vi "Load AFM Subpanel.vi"(0 "Ring in":refnum<vi>, 1 "Background Image":refnum<vi>, 3 "name or relative path":string, 5 "Inkscape File (.svg)":refnum<vi>, 7 "input cluster":T2, 9 "Subpanel":refnum<vi>, 11 "error in (no error)":errorcluster, 12 "Run":refnum<vi>, 14 "Abort":refnum<vi>) -> (6 "reference out":refnum<vi>, 15 "error out":errorcluster)   [LabVIEW 2013]
doc: "This VI opens an AFM subpanel."
uses:
  <vilib>/Analysis/Matrix/Datatypes/RealMatrix.ctl
  <vilib>/Analysis/Matrix/NI_Matrix.lvlib
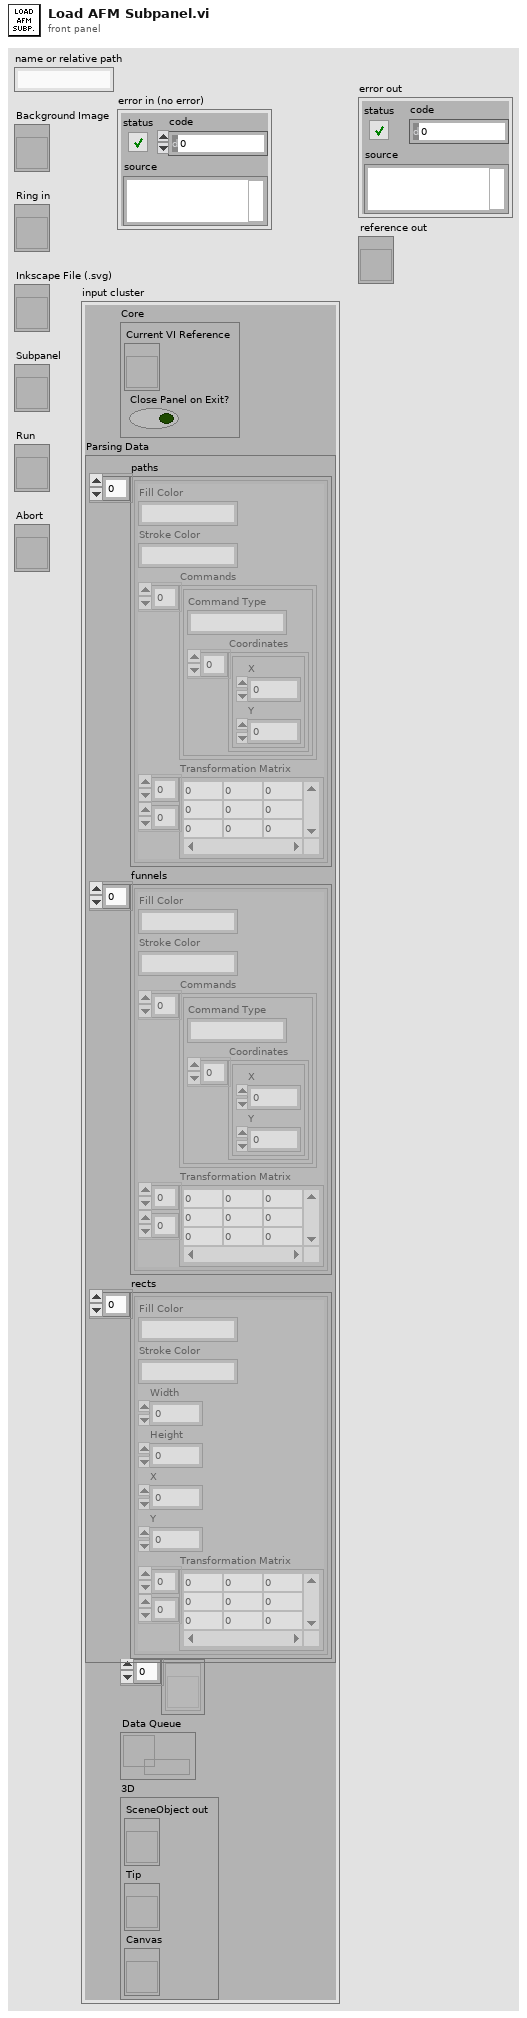
[diagram p1: front panel]
types:
  T1 = typedef "NI_Matrix.lvlib/RealMatrix.ctl" = dbl[][]
  T2 = cluster{"Core":cluster{"Current VI Reference":refnum<vi>, "Close Panel on Exit?":bool}, "Parsing Data":cluster{"paths":cluster{"Fill Color":string, "Stroke Color":string, "Commands":cluster{"Command Type":string, "Coordinates":cluster{"X":dbl, "Y":dbl}[]}[], "Transformation Matrix":T1}[], "funnels":cluster{"Fill Color":string, "Stroke Color":string, "Commands":cluster{"Command Type":string, "Coordinates":cluster{"X":dbl, "Y":dbl}[]}[], "Transformation Matrix":T1}[], "rects":cluster{"Fill Color":string, "Stroke Color":string, "Width":dbl, "Height":dbl, "X":dbl, "Y":dbl, "Transformation Matrix":T1}[]}, "Lithography Data":cluster{"Name":string, "Litho":cluster{"X":dbl, "Y":dbl, "Speed":dbl, "Voltage":dbl}[]}[], "VI Refs":refnum<vi>[], "Data Queue":refnum<queue>, "3D":cluster{"SceneObject out":refnum<vi>, "Tip":refnum<vi>, "Canvas":refnum<vi>}}
  T3 = cluster{"Name":string, "Litho":cluster{"X":dbl, "Y":dbl, "Speed":dbl, "Voltage":dbl}[]}[]
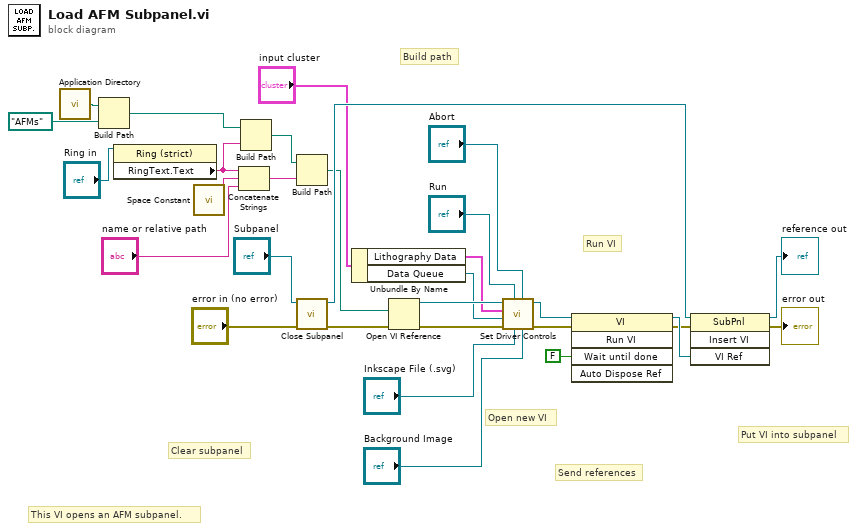
[diagram p0: block diagram]
diagram:
  # "This VI opens an AFM subpanel."
  # "Run VI"
  # "Put VI into subpanel"
  # "Send references"
  # "Open new VI"
  # "Clear subpanel"
  # "Build path"
  n1 = call <vilib>:"Application Directory.vi"() -> ("Application Directory"=w21:path)
  n2 = Build Path(base path=w21, name or relative path=path "AFMs" ("path")) -> (appended path=w23:path)
  n3 = property class="Ring (strict)"(reference="Ring in") -> ("RingText.Text"=w24:string)  [unwired: 1 in, 2 out]
  n4 = call <vilib>:"Space Constant.vi"() -> ("String"=w16:string)
  n5 = Concatenate Strings(w24, w16, "name or relative path") -> (w15:string)
  n6 = Build Path(base path=w23, name or relative path=w24) -> (appended path=w29:path)
  n7 = Build Path(base path=w29, name or relative path=w15) -> (appended path=w19:path)
  n8 = call "Close Subpanel.vi"("error in (no error)"="error in (no error)", "SubPanel in"="Subpanel") -> ("error out"=w30:errorcluster, "SubPanel out"=w27:refnum<vi>)  [unwired: 8 in]
  n9 = Unbundle By Name("input cluster") -> ("Lithography Data"=w9:T3, "Data Queue"=w8:refnum<queue>)
  n10 = Open VI Reference(vi path=w19, error in (no error)=w30) -> (vi reference=w11:refnum<vi>, error out=w12:errorcluster)  [unwired: 4 in]
  n11 = call "Set Driver Controls.vi"("Background Image"="Background Image", "Abort"="Abort", "Inkscape File (.svg)"="Inkscape File (.svg)", "Run"="Run", "error in (no error)"=w12, "Data Queue"=w8, "Lithography Data"=w9, "VI in"=w11) -> ("error out"=w13:errorcluster, "VI out"=w14:refnum<vi>)  [unwired: 2 in]
  n12 = invoke class="VI" method="Run VI"(reference=w14, error in=w13, "Wait until done"=FALSE ("Wait Until Done")) -> (reference out=w28:refnum<vi>, error out=w26:errorcluster)  [unwired: 2 in, 3 out]
  n13 = invoke class="SubPnl" method="Insert VI"(reference=w27, error in=w26, "VI Ref"=w28) -> (reference out=→"reference out":refnum<vi>, error out=→"error out":errorcluster)  [unwired: 1 in, 2 out]
